vi "Plot_Channels.vi"() -> (5 "Plug in titles":string[](array[string]), 7 "Plug in values":string[](array[string]))   [LabVIEW 2015]
uses:
  Globals/Meas_global.vi
panel:
  out "Size 2":i32
  out "Size 1":i32
  out "Size 0":i32
  in  "index 2":i32=3
  out "XY Graph":cluster{"Time (ms)":dbl[], "Eng Values":dbl[]}[](graph)
  in  "index 1":i32=1
  in  "index 0":i32
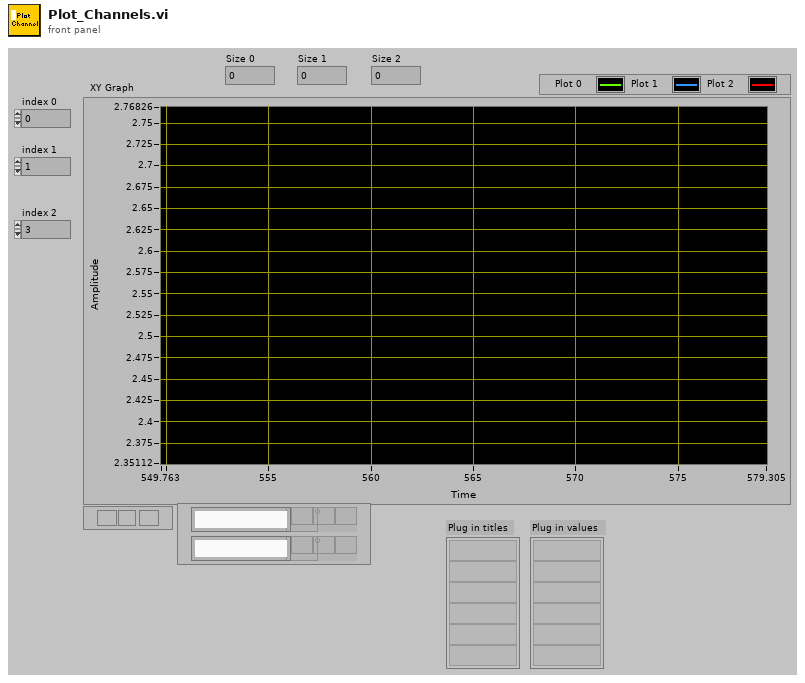
[diagram p1: front panel]
types:
  T1 = typedef "Time_Trace_Cluster.ctl" = cluster{"Weighting":dbl[], "Time (s)":dbl[], "Voltage":dbl[], "Eng Values":dbl[]}
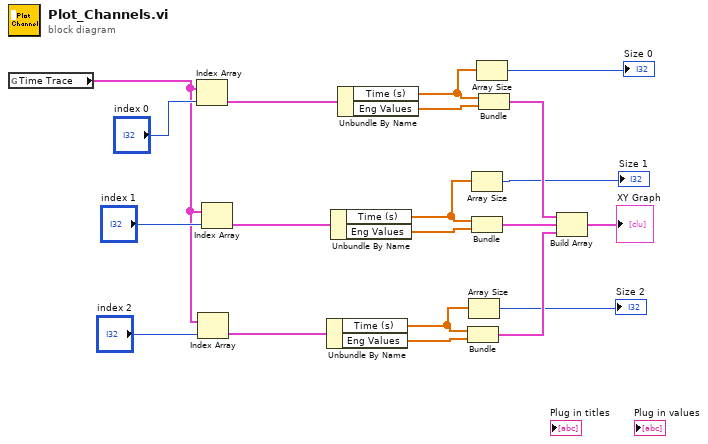
[diagram p0: block diagram]
diagram:
  n1 = global read "Meas_global.vi" "Time Trace"() -> (w4:T1[])
  n2 = Index Array(array=w4, index="index 0") -> (element=w1:T1)
  n3 = Index Array(array=w4, index="index 2") -> (element=w3:T1)
  n4 = Index Array(array=w4, index="index 1") -> (element=w2:T1)
  n5 = Unbundle By Name(w3) -> ("Time (s)"=w8:dbl[], "Eng Values"=w13:dbl[])
  n6 = Unbundle By Name(w2) -> ("Time (s)"=w9:dbl[], "Eng Values"=w17:dbl[])
  n7 = Unbundle By Name(w1) -> ("Time (s)"=w10:dbl[], "Eng Values"=w18:dbl[])
  n8 = Bundle("Time (s)"=w8, "Eng Values"=w13) -> (w11:cluster{"Time (s)":dbl[], "Eng Values":dbl[]})  [unwired: 1 in]
  n9 = Array Size(array=w8) -> (size(s)=→"Size 2":i32)
  n10 = Array Size(array=w9) -> (size(s)=→"Size 1":i32)
  n11 = Bundle("Time (s)"=w9, "Eng Values"=w17) -> (w16:cluster{"Time (s)":dbl[], "Eng Values":dbl[]})  [unwired: 1 in]
  n12 = Array Size(array=w10) -> (size(s)=→"Size 0":i32)
  n13 = Bundle("Time (s)"=w10, "Eng Values"=w18) -> (w15:cluster{"Time (s)":dbl[], "Eng Values":dbl[]})  [unwired: 1 in]
  n14 = Build Array(w15, w16, w11) -> (→"XY Graph":cluster{"Time (s)":dbl[], "Eng Values":dbl[]}[])
